vi "Get State Data.vi"(0 "SystemLink connection in":T2, 5 "state name":string, 11 "error in (no error)":errorcluster) -> (3 "attributes":T1, 4 "SystemLink connection out":T2, 8 "feeds":string[][](table), 10 "packages":string[][](table), 15 "error out":errorcluster)   [LabVIEW 2017, in "SystemLink_States_API.lvlib"]
doc: "Gets state data (attributes, feeds, packages) for the specified state name"
uses:
  SystemLink_States_API.lvlib
  _support/systemlink connection.ctl
  <vilib>/httpClient/ClientHandle.ctl
  52c1dc11-73db-4f81-b7ef-fb8e5fdf35ad.vi
  2be22946-5a21-4754-89c4-ff590a019e20.vi
  2f22416f-25c4-433a-99d4-052340b3f58f.vi
  <vilib>/JDP Science/JSONtext/Find Multiple Items.vi
  <vilib>/JDP Science/JSONtext/String Subset.vi
  <vilib>/JDP Science/JSONtext/support/Strip Quotes and Unescape.vi
  <vilib>/JDP Science/JSONtext/Parsing/Parse Full Path or Item Name.vi
  <vilib>/JDP Science/JSONtext/Offset/Find Item Locations by Path.vi
  <vilib>/JDP Science/JSONtext/support/Unescape JSON string.vi
  <vilib>/JDP Science/JSONtext/JSON text to Variant.vi
  <vilib>/httpClient/LabVIEWHTTPClient.lvlib
panel:
  out "state name out":string
  out "body":string
  out "headers":string
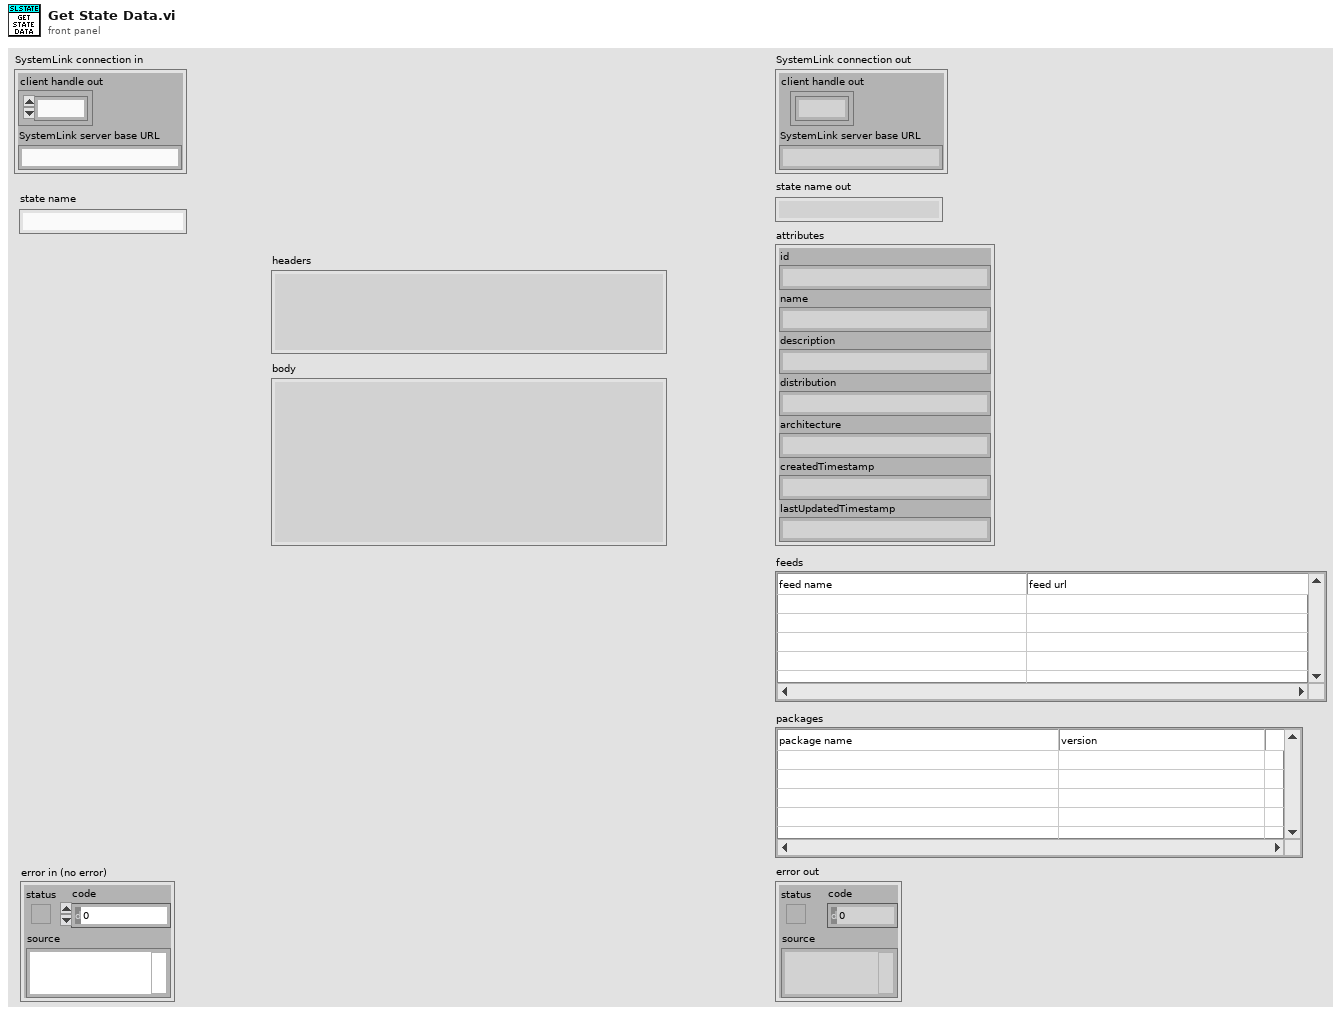
[diagram p1: front panel]
types:
  T1 = cluster{"id":string, "name":string, "description":string, "distribution":string, "architecture":string, "createdTimestamp":string, "lastUpdatedTimestamp":string}
  T2 = typedef "SystemLink_States_API.lvlib/systemlink connection.ctl" = cluster{"client handle out":T3, "SystemLink server base URL":string}
  T3 = typedef "LabVIEWHTTPClient.lvlib/ClientHandle.ctl" = refnum<k1>
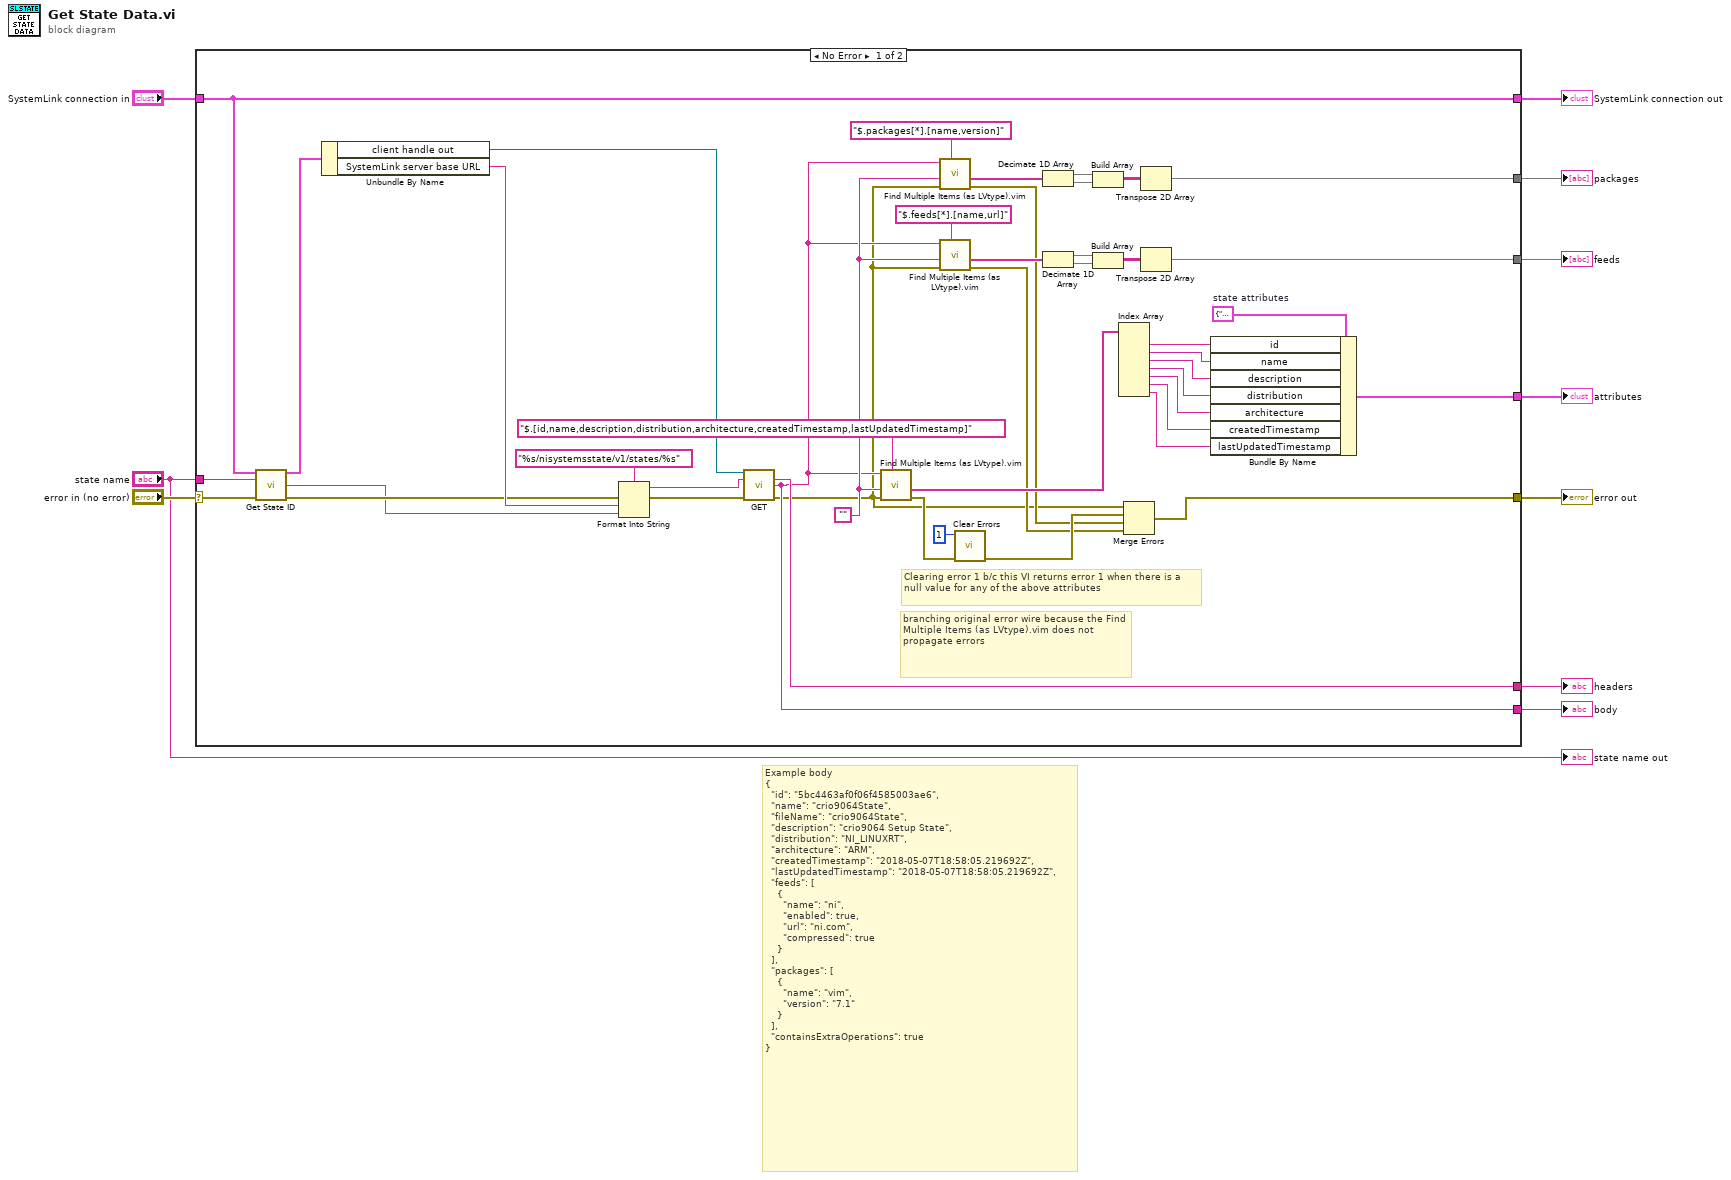
[diagram p0: block diagram]
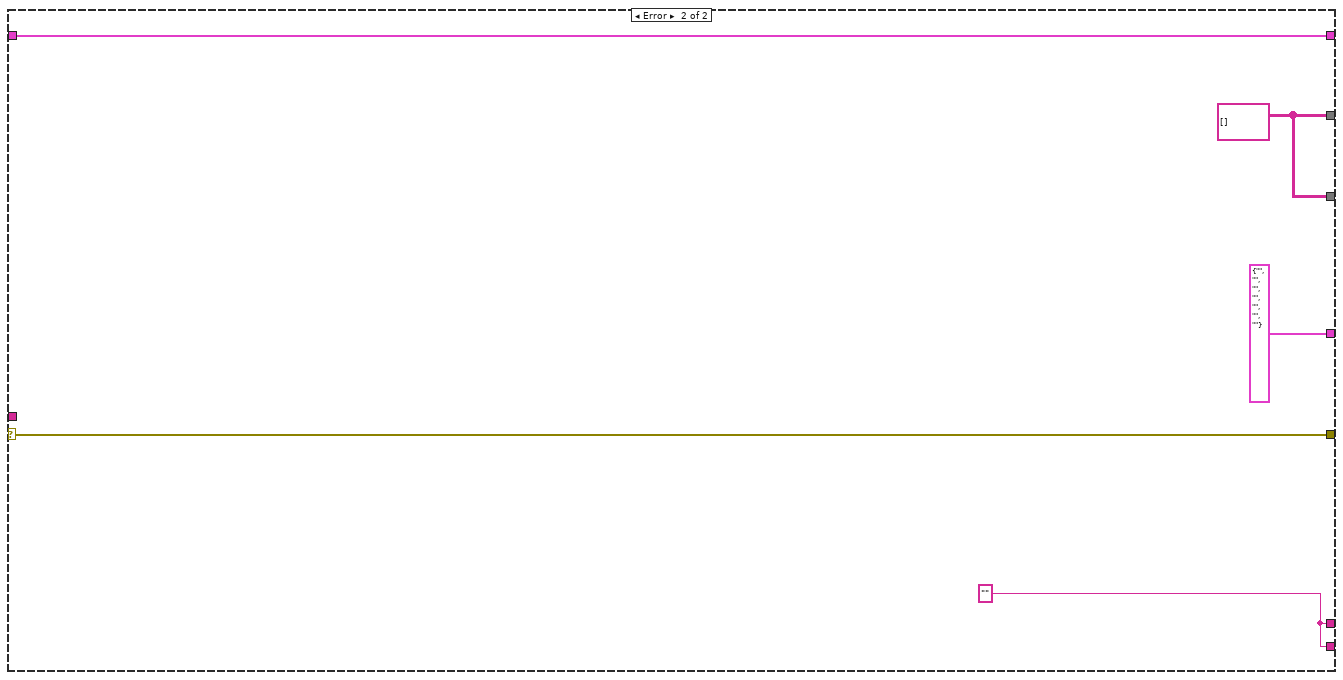
[diagram p2: hidden frame]
diagram:
  # "Example body\n{\n  \"id\": \"5bc4463af0f06f4585003ae6\",\n  \"name\": \"crio9064State\",\n  \"fileName\": \"crio9064State\",\n  \"description\": \"crio9064 Setup State\",\n  \"distribution\": \"NI_LINUXRT\",\n  \"architecture\": \"ARM\",\n  \"createdTimestamp\": \"2018-05-07T18:58:05.219692Z\",\n  \"lastUpdatedTimestamp\": \"2018-05-07T18:58:05.219692Z\",\n  \"feeds\": [\n    {\n      \"name\": \"ni\",\n      \"enabled\": true,\n      \"url\": \"ni.com\",\n      \"compressed\": true\n    }\n  ],\n  \"packages\": [\n    {\n      \"name\": \"vim\",\n      \"version\": \"7.1\"\n    }\n  ],\n  \"containsExtraOperations\": true\n}"
  n1 = case shown="No Error" "error in (no error)" {
    selector: "error in (no error)" -> [w45 w59]
    tunnel: "SystemLink connection in" -> [w43 w57]
    tunnel: [w47 w59] -> w8
    tunnel: [w34 w58] -> w7
    tunnel: [w48 w58] -> w6
    tunnel: [w43 w57] -> w5
    tunnel: "state name" -> [w41 _]
    tunnel: [w16 T1 {"id"="", "name"="", "description"="", "distribution"="", "architecture"="", "createdTimestamp"="", "lastUpdatedTimestamp"=""} ("state attributes")] -> w3
    tunnel: [w15 w56] -> w2
    tunnel: [w14 w56] -> w1
    frame No Error {
      w25 = T1 {"id"="", "name"="", "description"="", "distribution"="", "architecture"="", "createdTimestamp"="", "lastUpdatedTimestamp"=""}  # state attributes
      w35 = ""
      # "Clearing error 1 b/c this VI returns error 1 when there is a null value for any of the above attributes"
      # "branching original error wire because the Find Multiple Items (as LVtype).vim does not propagate errors"
      n2 = call "Get State ID.vi"("SystemLink connection in"=w43, "state name"=w41, "error in (no error)"=w45) -> ("SystemLink connection out"=w42:T2, "state ID"=w40:string, "error out"=w44:errorcluster)  [unwired: 9 in, 1 out]
      n3 = Unbundle By Name(w42) -> ("client handle out"=w52:T3, "SystemLink server base URL"=w49:string)
      n4 = Format Into String(format string="%s/nisystemsstate/v1/states/%s", error in=w44, w49, w40) -> (resulting string=w53:string, error out=w51:errorcluster)  [unwired: 1 in]
      n5 = call <vilib>:"GET.vi"("client handle"=w52, "url"=w53, "error in (no error)"=w51) -> ("headers"=w48:string, "body"=w34:string, "error out"=w11:errorcluster)  [unwired: 9 in, 1 out]
      n6 = call "Find Multiple Items (as LVtype).vim"("$Path or Item Name"="$.[id,name,description,distribution,architecture,createdTimestamp,lastUpdatedTimestamp]", "error in (no error)"=w11, "Data Type and Default Value"=w35, "JSON"=w34) -> ("error out"=w46:errorcluster, "Array of Data"=w24:string[])  [unwired: 4 in, 2 out]
      n7 = call "Find Multiple Items (as LVtype).vim"("$Path or Item Name"="$.packages[*].[name,version]", "error in (no error)"=w11, "Data Type and Default Value"=w35, "JSON"=w34) -> ("error out"=w13:errorcluster, "Array of Data"=w33:string[])  [unwired: 4 in, 2 out]
      n8 = call "Find Multiple Items (as LVtype).vim"("$Path or Item Name"="$.feeds[*].[name,url]", "error in (no error)"=w11, "Data Type and Default Value"=w35, "JSON"=w34) -> ("error out"=w12:errorcluster, "Array of Data"=w26:string[])  [unwired: 4 in, 2 out]
      n9 = call <vilib>:"Clear Errors.vi"("error in (no error)"=w46, "specific error code to clear (0: all)"=1) -> ("error out"=w38:errorcluster)  [unwired: 4 in, 1 out]
      n10 = Decimate 1D Array(w33) -> (w32:string[], w31:string[])
      n11 = Decimate 1D Array(w26) -> (w27:string[], w28:string[])
      n12 = Build Array(w32, w31) -> (w30:string[][])
      n13 = Build Array(w27, w28) -> (w29:string[][])
      n14 = Index Array(array=w24) -> (element #1=w23:string, element #2=w22:string, element #3=w21:string, element #4=w20:string, element #5=w19:string, element #6=w18:string, element #7=w17:string)  [unwired: 7 in]
      n15 = Merge Errors(w11, w38, w13, w12) -> (w47:errorcluster)
      n16 = Transpose 2D Array(2D array=w30) -> (transposed array=w15:string[][])
      n17 = Transpose 2D Array(2D array=w29) -> (transposed array=w14:string[][])
      n18 = Bundle By Name(cluster=w25, "id"=w23, "name"=w22, "description"=w21, "distribution"=w20, "architecture"=w19, "createdTimestamp"=w18, "lastUpdatedTimestamp"=w17) -> (w16:T1)
    }
    frame Error {
      w56 = string[][] []
      w58 = "" ("headers")
    }
  }
  "error out" <- w8
  "SystemLink connection out" <- w5
  "headers" <- w6
  "body" <- w7
  "feeds" <- w1
  "packages" <- w2
  "attributes" <- w3
  "state name out" <- "state name"
